vi "WritePRN.vi"(8 "error in (no error)":errorcluster, 9 "2D Data":sgl[][](array[numeric]), 10 "1D Data":sgl[](array[numeric]), 11 "Data Path (Send to Mathcad)":path) -> (0 "error out":errorcluster, 3 "Data Path(String)":string)   [LabVIEW 2015]
doc: "Sends a 1-D or 2-D array to a file that Mathcad can Read. Use the READPRN function to read the data file in Mathcad.\n\nInputs\nData Path(Send to Mathcad)- (Path Data type)- Full path to the data file\n2D Data- The 2D data contains the single-precision numbers the VI writes to the file if 1D data is not wired or is empty. \n1D Data- The 1D data contains the single-precision numbers the VI writes to the file\nOutputs\nData Path (String) - (String Data type)- This is the String data type of the Data Path input. You can use this output to write a string variable to Mathcad to indicate the location of the data\nError Out- Erro Cluster out."
uses:
  <vilib>/Utility/file.llb/Write To Spreadsheet File (DBL).vi
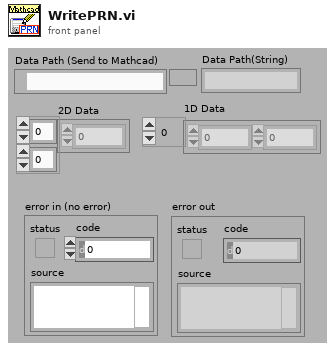
[diagram p1: front panel]
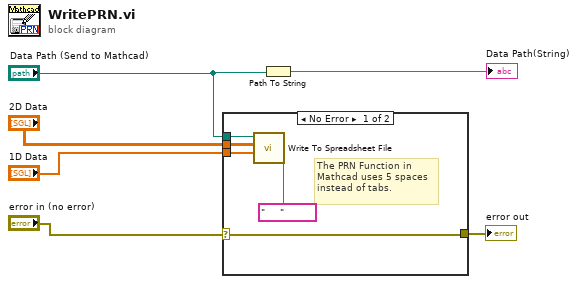
[diagram p0: block diagram]
diagram:
  n1 = case shown="No Error" "error in (no error)" {
    selector: "error in (no error)" -> [w8 w12]
    tunnel: "2D Data" -> [w11 _]
    tunnel: "Data Path (Send to Mathcad)" -> [w10 _]
    tunnel: [w8 w12] -> w6
    tunnel: "1D Data" -> [w7 _]
    frame No Error {
      # "The PRN Function in\nMathcad uses 5 spaces\ninstead of tabs."
      n2 = call-poly <vilib>:"Write To Spreadsheet File.vi"("delimiter (\\t)"="     " ("delimiter (Tab)"), "1D data"=w7, "2D data"=w11, "file path (dialog if empty)"=w10) -> ()  [unwired: 4 in, 1 out]
    }
    frame Error {
    }
  }
  "error out" <- w6
  n3 = Path To String(path="Data Path (Send to Mathcad)") -> (string=→"Data Path(String)":string)
